vi "Play.vi"(8 "error in (no error)":errorcluster, 10 "Sound":refnum<class "Sound.lvclass">, 11 "Sound Visualizer":refnum<class "Sound Visualizer.lvclass">) -> (0 "error out":errorcluster, 3 "Sound Player out":refnum<class "Sound Visualizer.lvclass">)   [LabVIEW 2010, in "Sound Visualizer.lvclass"]
doc: "Play a sound on the visualizer."
uses:
  Sound Visualizer.lvclass
  Sound/Sound.lvclass
  Sound Visualizer.lvclass/Sound Visualizer.ctl
  Visualizer/Visualizer.lvlib
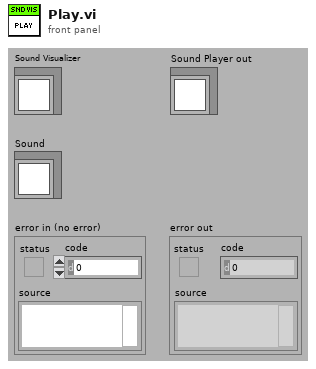
[diagram p1: front panel]
types:
  T1 = typedef "Visualizer.lvlib/Visualizer Type ID.ctl" = u32
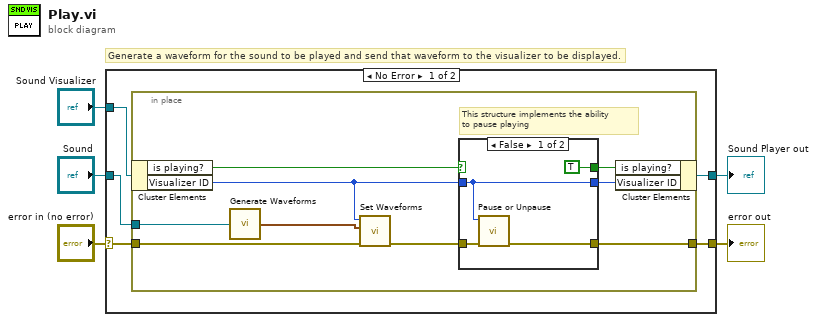
[diagram p0: block diagram]
diagram:
  # "Generate a waveform for the sound to be played and send that waveform to the visualizer to be displayed."
  n1 = case shown="No Error" "error in (no error)" {
    selector: "error in (no error)" -> [w9 w28]
    tunnel: [w7 w28] -> w4
    tunnel: "Sound Visualizer" -> [w8 w27]
    tunnel: "Sound" -> [w10 _]
    tunnel: [w6 w27] -> w1
    frame No Error {
      n2 = in-place {
        in-place-border: w10 -> [w19]
        in-place-border: w9 -> [w17]
        in-place-border: [w13] -> w7
        # "This structure implements the ability \nto pause playing"
        n3 = in-place-cluster #1(w8) -> ("is playing?"=w14:bool, "Visualizer ID"=w15:T1)
        n4 = call "Generate Waveforms.vi"("Sound.lvclass"=w19) -> ("Waveforms"=w18:waveform(dbl)[])
        n5 = call "Set Waveforms.vi"("error in (no error)"=w17, "Waveforms"=w18, "Visualizer ID"=w15) -> ("error out"=w16:errorcluster)  [unwired: 8 in]
        n6 = case shown="False" w14 {
          selector: w14 -> [_ w25]
          tunnel: w16 -> [w23 w26]
          tunnel: w15 -> [w20 w24]
          tunnel: [w22 w26] -> w13
          tunnel: [TRUE w25] -> w12
          tunnel: [w20 w24] -> w11
          frame False {
            n7 = call "Pause or Unpause.vi"("error in (no error)"=w23, "Visualizer ID"=w20) -> ("error out"=w22:errorcluster)  [unwired: 9 in]
          }
          frame True {
          }
        }
        n8 = in-place-cluster #1("is playing?"=w12, "Visualizer ID"=w11) -> (w6:refnum<class "Sound Visualizer.lvclass">)
      }
    }
    frame Error {
    }
  }
  "error out" <- w4
  "Sound Player out" <- w1
